vi "[nc] Piece-specific modifications.vi"(8 "error in (no error)":errorcluster, 10 "Position in":refnum<class "Position.lvclass">, 11 "Piece in":refnum<class "Piece.lvclass">) -> (0 "error out":errorcluster, 2 "Position out":refnum<class "Position.lvclass">, 3 "Piece out":refnum<class "Piece.lvclass">)   [LabVIEW 2016]
uses:
  Piece.lvclass
  Position/Position.lvclass
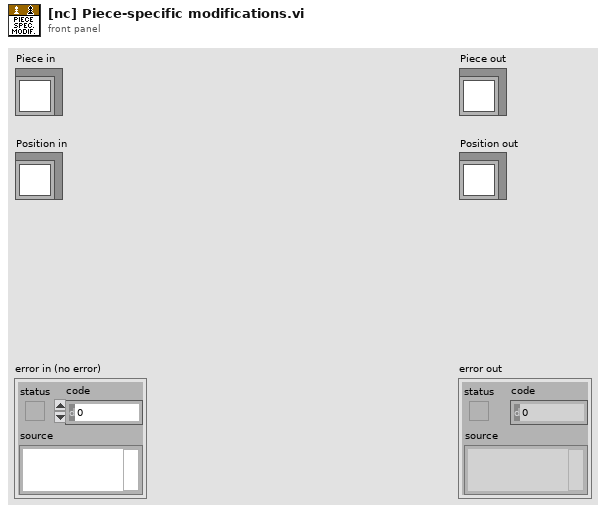
[diagram p1: front panel]
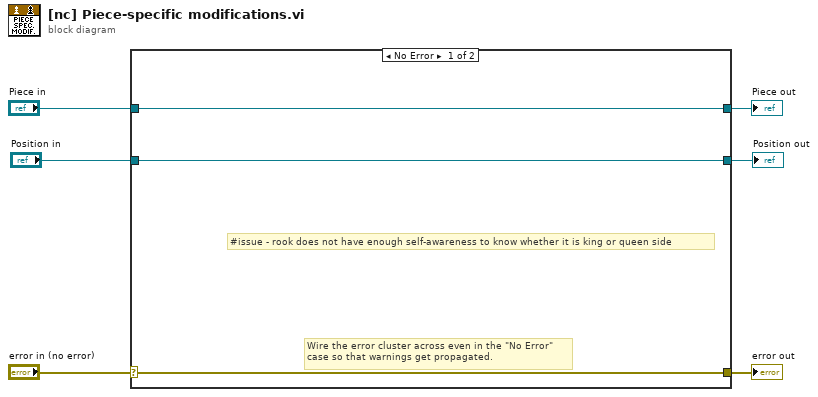
[diagram p0: block diagram]
diagram:
  n1 = case shown="No Error" "error in (no error)" {
    selector: "error in (no error)" -> [w8 w12]
    tunnel: [w8 w12] -> w5
    tunnel: [w9 w11] -> w3
    tunnel: "Piece in" -> [w9 w11]
    tunnel: [w7 w10] -> w2
    tunnel: "Position in" -> [w7 w10]
    frame No Error {
      # "#issue - rook does not have enough self-awareness to know whether it is king or queen side"
      # "Wire the error cluster across even in the \"No Error\"\ncase so that warnings get propagated."
    }
    frame Error {
    }
  }
  "error out" <- w5
  "Piece out" <- w3
  "Position out" <- w2
